vi "State_machine.vi"() -> ()   [LabVIEW 2022 SP3]
uses:
  SM_States.ctl
  SM_Data.ctl
panel:
  in  "SM_Data":T1
  in  "Stop":bool
  in  "Reset":bool
  out "Numbers":string
  in  "OK Button 10":bool
  in  "OK Button 9":bool
  in  "OK Button 8":bool
  in  "OK Button 7":bool
  in  "OK Button 6":bool
  in  "OK Button 5":bool
  in  "OK Button 4":bool
  in  "OK Button 3":bool
  in  "OK Button 2":bool
  in  "OK Button":bool
  in  "SM_States":T2
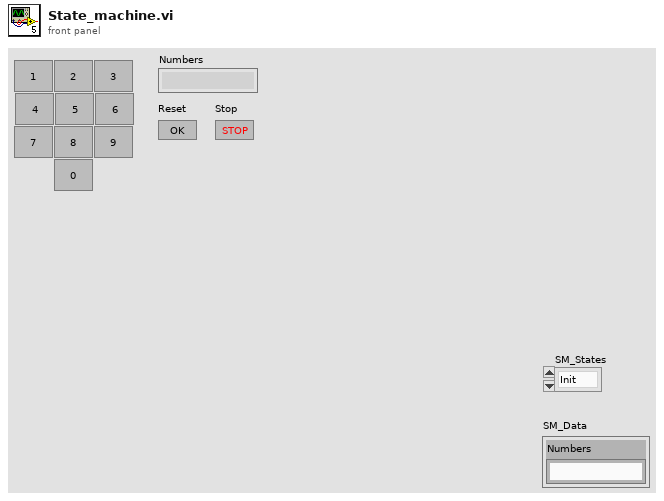
[diagram p1: front panel]
types:
  T1 = typedef "SM_Data.ctl" = cluster{"Numbers":string}
  T2 = typedef "SM_States.ctl" = enum16{"Init", "Stop", "Reset", "Idle"}
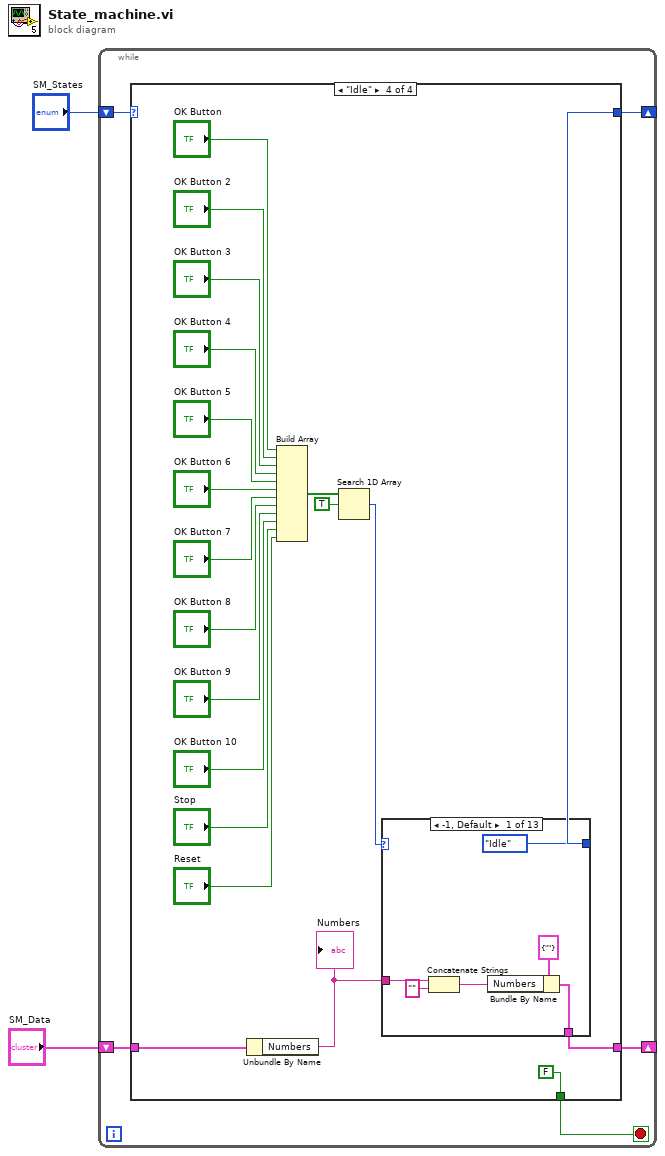
[diagram p0: block diagram]
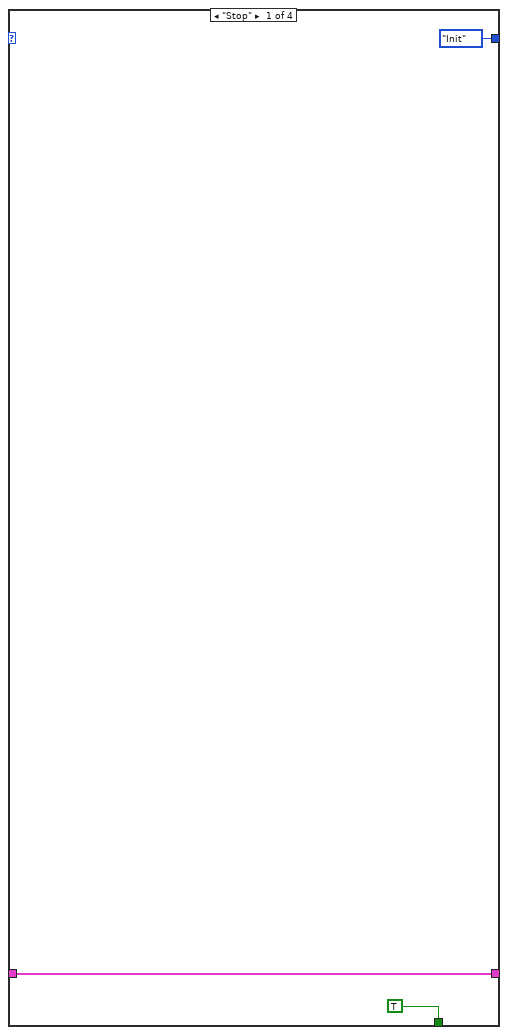
[diagram p2: hidden frame]
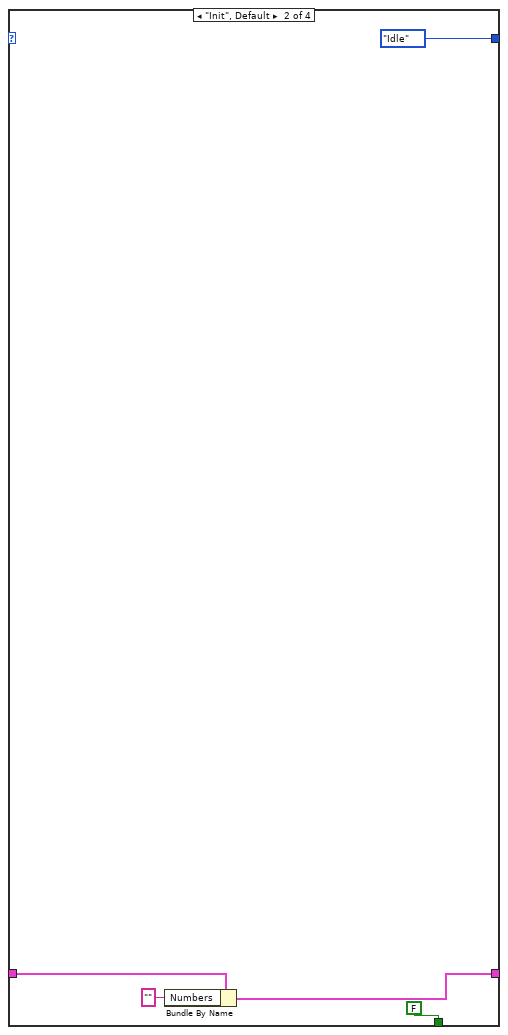
[diagram p3: hidden frame]
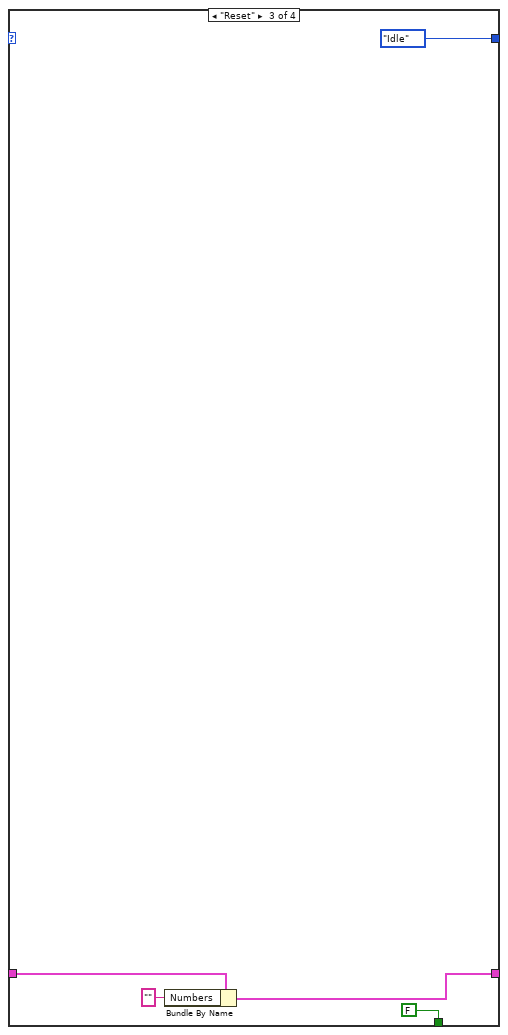
[diagram p4: hidden frame]
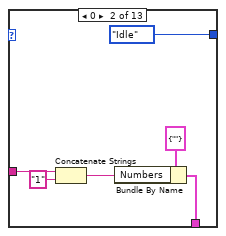
[diagram p5: hidden frame]
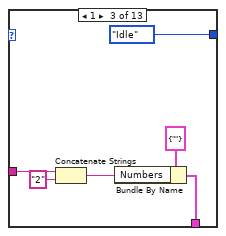
[diagram p6: hidden frame]
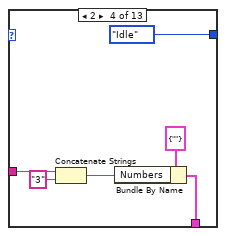
[diagram p7: hidden frame]
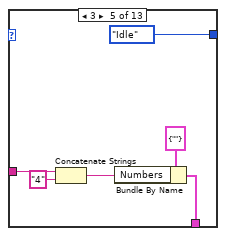
[diagram p8: hidden frame]
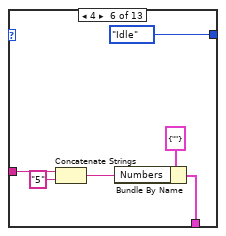
[diagram p9: hidden frame]
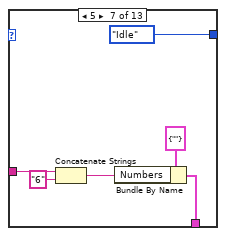
[diagram p10: hidden frame]
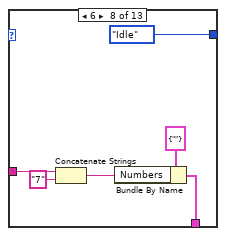
[diagram p11: hidden frame]
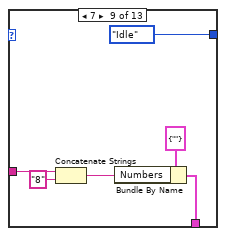
[diagram p12: hidden frame]
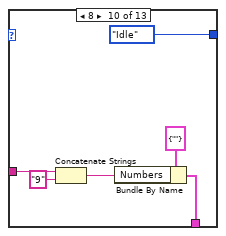
[diagram p13: hidden frame]
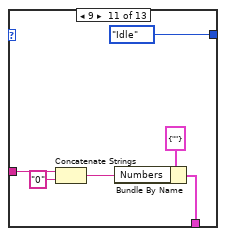
[diagram p14: hidden frame]
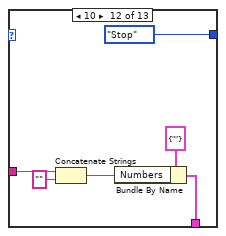
[diagram p15: hidden frame]
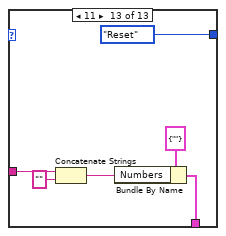
[diagram p16: hidden frame]
diagram:
  n1 = while {
    shift-right: [w6] -> _
    shift-left: "SM_States" -> [w7]
    shift-right: [w4] -> _
    shift-left: "SM_Data" -> [w5]
    stop <- w3 stop-if-true
    n2 = case shown="\"Idle\"" w7 {
      tunnel: [SM_States."Init" ("SM_States") SM_States."Idle" ("SM_States") SM_States."Idle" ("SM_States") w23] -> w6
      tunnel: w5 -> [w9 w14 w19 w25]
      tunnel: [w9 w13 w18 w21] -> w4
      tunnel: [TRUE FALSE FALSE FALSE] -> w3
      frame "Stop" {
      }
      frame "Init", Default {
        n3 = Bundle By Name(cluster=w14, "Numbers"="") -> (w13:T1)
      }
      frame "Reset" {
        n4 = Bundle By Name(cluster=w19, "Numbers"="") -> (w18:T1)
      }
      frame "Idle" {
        n5 = Unbundle By Name(w25) -> ("Numbers"=w22:string)
        "Numbers" <- w22
        n6 = Build Array("OK Button", "OK Button 2", "OK Button 3", "OK Button 4", "OK Button 5", "OK Button 6", "OK Button 7", "OK Button 8", "OK Button 9", "OK Button 10", "Stop", "Reset") -> (w28:bool[])
        n7 = Search 1D Array(1D array=w28, element=TRUE) -> (index of element=w26:i32)  [unwired: 1 in]
        n8 = case shown="-1, Default" w26 {
          tunnel: [SM_States."Idle" ("SM_States") SM_States."Idle" ("SM_States") SM_States."Idle" ("SM_States") SM_States."Idle" ("SM_States") SM_States."Idle" ("SM_States") SM_States."Idle" ("SM_States") SM_States."Idle" ("SM_States") SM_States."Idle" ("SM_States") SM_States."Idle" ("SM_States") SM_States."Idle" ("SM_States") SM_States."Idle" ("SM_States") SM_States."Stop" ("SM_States") SM_States."Reset" ("SM_States")] -> w23
          tunnel: w22 -> [w45 w51 w57 w63 w69 w75 w81 w87 w93 w99 w105 w111 w117]
          tunnel: [w41 w47 w53 w59 w65 w71 w77 w83 w89 w95 w101 w107 w113] -> w21
          frame -1, Default {
            n9 = Concatenate Strings(w45, "" ("string")) -> (w42:string)
            n10 = Bundle By Name(cluster=T1 {"Numbers"=""} ("SM_Data"), "Numbers"=w42) -> (w41:T1)
          }
          frame 0 {
            n11 = Concatenate Strings(w51, "1" ("string")) -> (w48:string)
            n12 = Bundle By Name(cluster=T1 {"Numbers"=""} ("SM_Data"), "Numbers"=w48) -> (w47:T1)
          }
          frame 1 {
            n13 = Concatenate Strings(w57, "2" ("string")) -> (w54:string)
            n14 = Bundle By Name(cluster=T1 {"Numbers"=""} ("SM_Data"), "Numbers"=w54) -> (w53:T1)
          }
          frame 2 {
            n15 = Concatenate Strings(w63, "3" ("string")) -> (w60:string)
            n16 = Bundle By Name(cluster=T1 {"Numbers"=""} ("SM_Data"), "Numbers"=w60) -> (w59:T1)
          }
          frame 3 {
            n17 = Concatenate Strings(w69, "4" ("string")) -> (w66:string)
            n18 = Bundle By Name(cluster=T1 {"Numbers"=""} ("SM_Data"), "Numbers"=w66) -> (w65:T1)
          }
          frame 4 {
            n19 = Concatenate Strings(w75, "5" ("string")) -> (w72:string)
            n20 = Bundle By Name(cluster=T1 {"Numbers"=""} ("SM_Data"), "Numbers"=w72) -> (w71:T1)
          }
          frame 5 {
            n21 = Concatenate Strings(w81, "6" ("string")) -> (w78:string)
            n22 = Bundle By Name(cluster=T1 {"Numbers"=""} ("SM_Data"), "Numbers"=w78) -> (w77:T1)
          }
          frame 6 {
            n23 = Concatenate Strings(w87, "7" ("string")) -> (w84:string)
            n24 = Bundle By Name(cluster=T1 {"Numbers"=""} ("SM_Data"), "Numbers"=w84) -> (w83:T1)
          }
          frame 7 {
            n25 = Concatenate Strings(w93, "8" ("string")) -> (w90:string)
            n26 = Bundle By Name(cluster=T1 {"Numbers"=""} ("SM_Data"), "Numbers"=w90) -> (w89:T1)
          }
          frame 8 {
            n27 = Concatenate Strings(w99, "9" ("string")) -> (w96:string)
            n28 = Bundle By Name(cluster=T1 {"Numbers"=""} ("SM_Data"), "Numbers"=w96) -> (w95:T1)
          }
          frame 9 {
            n29 = Concatenate Strings(w105, "0" ("string")) -> (w102:string)
            n30 = Bundle By Name(cluster=T1 {"Numbers"=""} ("SM_Data"), "Numbers"=w102) -> (w101:T1)
          }
          frame 10 {
            n31 = Concatenate Strings(w111, "" ("string")) -> (w108:string)
            n32 = Bundle By Name(cluster=T1 {"Numbers"=""} ("SM_Data"), "Numbers"=w108) -> (w107:T1)
          }
          frame 11 {
            n33 = Concatenate Strings(w117, "" ("string")) -> (w114:string)
            n34 = Bundle By Name(cluster=T1 {"Numbers"=""} ("SM_Data"), "Numbers"=w114) -> (w113:T1)
          }
        }
      }
    }
  }
